vi "GeneratorT.vi"(4 "tetha_o_pp":dbl, 5 "a0":dbl, 6 "tetha_f_p":dbl, 7 "a0":dbl, 8 "tetha_o_p":dbl, 9 "a0":dbl, 10 "tetha_f_pp":dbl, 11 "a0":dbl) -> (3 "Cluster":T1)   [LabVIEW 2018]
uses:
  <vilib>/Analysis/baseanly.llb/Real Inverse Matrix.vi
  <vilib>/Analysis/Matrix/Numeric/Conversions/Array To Matrix - RA2.vi
  <vilib>/Analysis/Matrix/Numeric/Multiply/Multiply - RM,RM.vi
  <vilib>/Analysis/NI_AALBase.lvlib
  <vilib>/Analysis/Matrix/NI_Matrix.lvlib
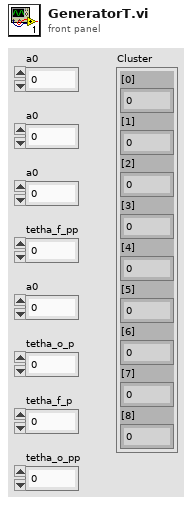
[diagram p1: front panel]
types:
  T1 = cluster{"[0]":dbl, "[1]":dbl, "[2]":dbl, "[3]":dbl, "[4]":dbl, "[5]":dbl, "[6]":dbl, "[7]":dbl, "[8]":dbl}
  T2 = typedef "NI_Matrix.lvlib/RealMatrix.ctl" = dbl[][]
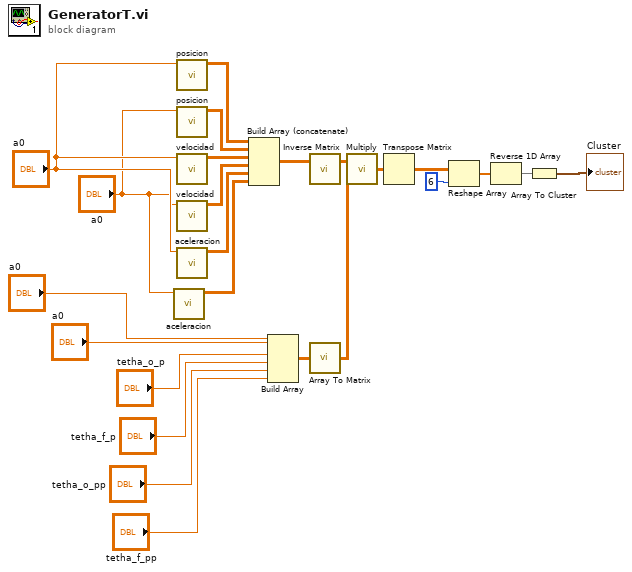
[diagram p0: block diagram]
diagram:
  n1 = call "aceleracion.vi"("a0"="a0") -> ("Real Matrix"=w22:T2)  [unwired: 10 in]
  n2 = call "posicion.vi"("a0"="a0") -> ("Real Matrix"=w1:T2)  [unwired: 10 in]
  n3 = call "posicion.vi"("a0"="a0") -> ("Real Matrix"=w19:T2)  [unwired: 10 in]
  n4 = call "velocidad.vi"("a0"="a0") -> ("Real Matrix"=w2:T2)  [unwired: 10 in]
  n5 = call "velocidad.vi"("a0"="a0") -> ("Real Matrix"=w20:T2)  [unwired: 10 in]
  n6 = call "aceleracion.vi"("a0"="a0") -> ("Real Matrix"=w3:T2)  [unwired: 10 in]
  n7 = Build Array (concatenate) ("Build Matrix")(w1, w19, w2, w20, w3, w22) -> (w15:T2)
  n8 = Build Array("a0", "a0", "tetha_o_p", "tetha_f_p", "tetha_o_pp", "tetha_f_pp") -> (w4:T2)
  n9 = call-poly <vilib>:"Inverse Matrix.vi"("Input Matrix"=w15) -> ("Inverse Matrix"=w14:T2)  [unwired: 1 in, 1 out]
  n10 = call-poly <vilib>:"Array To Matrix.vi"("Real 2D Array"=w4) -> ("Real Matrix"=w5:T2)
  n11 = call-poly <vilib>:"Multiply.vi"("Real Matrix B"=w5, "Real Matrix A"=w14) -> ("A * B"=w12:T2)
  n12 = Transpose Matrix(1:w12) -> (0:w13:T2)
  n13 = Reshape Array(w13, 6 ("dimension size")) -> (w16:dbl[])
  n14 = Reverse 1D Array(array=w16) -> (reversed array=w17:dbl[])
  n15 = Array To Cluster(array=w17) -> (cluster=→"Cluster":T1)
